vi "Check Limit&TestName Between STDF For Different Tester.vi"(7 "Result Length Array":i32[](array[numeric]), 8 "error in (no error)":errorcluster, 9 "Test Name Array":string[](array[string]), 10 "Low Limit Array":dbl[](array[numeric]), 11 "High Limit Array":dbl[](array[numeric])) -> (0 "error out":errorcluster, 3 "Test Data Out":T1)   [LabVIEW 2018, in "STDF File Parser.lvclass"]
uses:
  STDF File Parser.lvclass
  TestDataMgr/Typedefs/Test Data All.ctl
  TestDataMgr/Typedefs/Test Limits.ctl
  TestDataMgr/Typedefs/Test Raw Data.ctl
  <vilib>/Utility/error.llb/Error Cluster From Error Code.vi
  <vilib>/ErrorRing/Error Ring.xnode
  TestDataMgr/TestDataMgr.lvclass
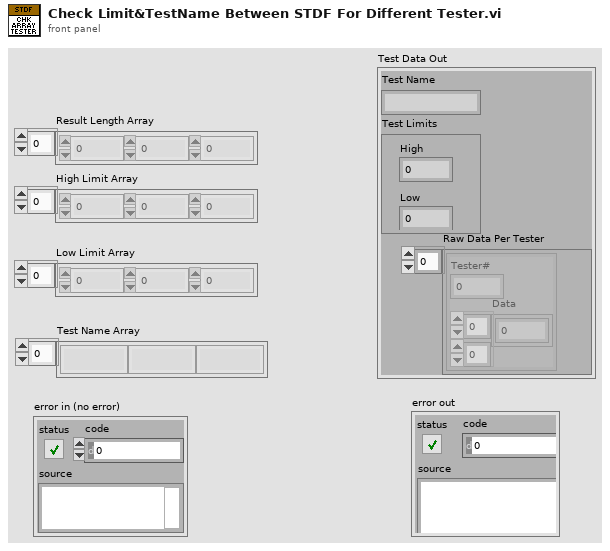
[diagram p1: front panel]
types:
  T1 = typedef "TestDataMgr.lvclass/Test Data All.ctl" = cluster{"Test Name":string, "Test Limits":T2, "Raw Data Per Tester":T3[]}
  T2 = typedef "TestDataMgr.lvclass/Test Limits.ctl" = cluster{"High":dbl, "Low":dbl}
  T3 = typedef "TestDataMgr.lvclass/Test Raw Data.ctl" = cluster{"Data":dbl[][], "Tester#":u8}
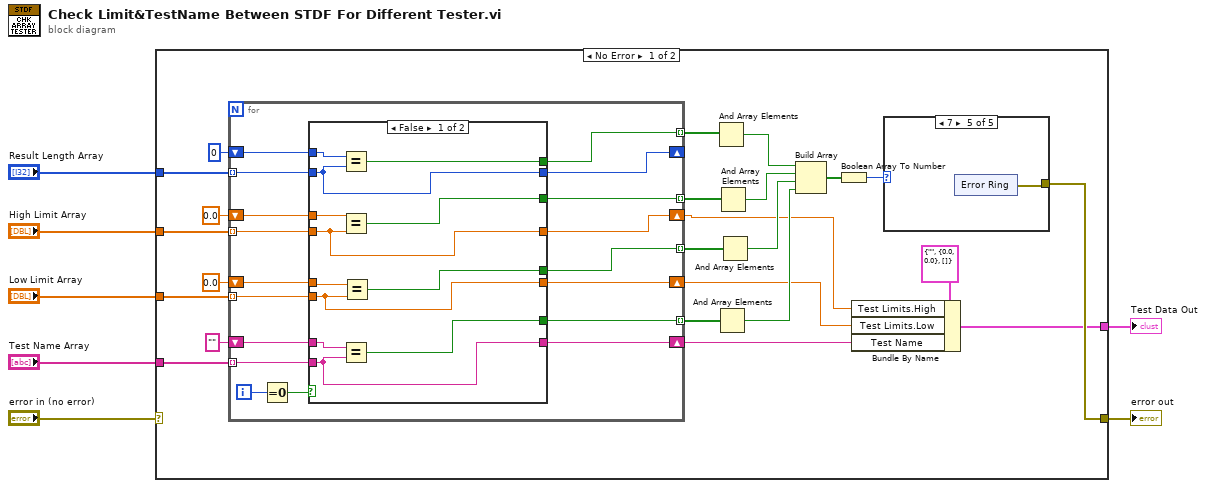
[diagram p0: block diagram]
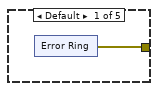
[diagram p2: hidden frame]
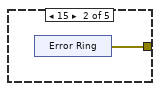
[diagram p3: hidden frame]
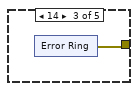
[diagram p4: hidden frame]
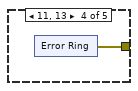
[diagram p5: hidden frame]
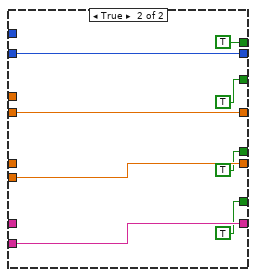
[diagram p6: hidden frame]
diagram:
  n1 = case shown="No Error" "error in (no error)" {
    selector: "error in (no error)" -> [_ w96]
    tunnel: "High Limit Array" -> [w31 _]
    tunnel: "Low Limit Array" -> [w30 _]
    tunnel: "Test Name Array" -> [w29 _]
    tunnel: "Result Length Array" -> [w25 _]
    tunnel: [w13 w96] -> w3
    tunnel: [w8 _] -> w1
    frame No Error {
      n2 = for {
        tunnel: w31 -> [w68] mode=indexing
        tunnel: w30 -> [w70] mode=indexing
        tunnel: w29 -> [w73] mode=indexing
        shift-right: [w72] -> w9
        shift-left: "" ("String") -> [w71]
        shift-right: [w69] -> w10
        shift-left: 0.0 ("High Limit Array") -> [w65]
        shift-right: [w67] -> w11
        shift-left: 0.0 ("High Limit Array") -> [w66]
        tunnel: w25 -> [w64] mode=indexing
        shift-right: [w63] -> _
        shift-left: 0 ("High Limit Array") -> [w62]
        tunnel: [w61] -> w23 mode=indexing
        tunnel: [w60] -> w22 mode=indexing
        tunnel: [w59] -> w21 mode=indexing
        tunnel: [w58] -> w20 mode=indexing
        i -> [w75]
        n3 = Equal To 0?(x=w75) -> (x = 0?=w74:bool)
        n4 = case shown="False" w74 {
          tunnel: w73 -> [w80 w95]
          tunnel: [w80 w95] -> w72
          tunnel: w71 -> [w84 _]
          tunnel: w70 -> [w81 w94]
          tunnel: [w81 w94] -> w69
          tunnel: [w82 w93] -> w67
          tunnel: w68 -> [w82 w93]
          tunnel: w66 -> [w87 _]
          tunnel: w65 -> [w85 _]
          tunnel: w64 -> [w83 w92]
          tunnel: [w83 w92] -> w63
          tunnel: w62 -> [w86 _]
          tunnel: [w79 TRUE] -> w61
          tunnel: [w76 TRUE] -> w60
          tunnel: [w78 TRUE] -> w59
          tunnel: [w77 TRUE] -> w58
          frame False {
            n5 = Equal?(x=w86, y=w83) -> (x = y?=w79:bool)
            n6 = Equal?(x=w87, y=w82) -> (x = y?=w76:bool)
            n7 = Equal?(x=w84, y=w80) -> (x = y?=w77:bool)
            n8 = Equal?(x=w85, y=w81) -> (x = y?=w78:bool)
          }
          frame True {
          }
        }
      }
      n9 = And Array Elements(Boolean array=w23) -> (logical AND=w19:bool)
      n10 = And Array Elements(Boolean array=w20) -> (logical AND=w16:bool)
      n11 = And Array Elements(Boolean array=w22) -> (logical AND=w18:bool)
      n12 = And Array Elements(Boolean array=w21) -> (logical AND=w17:bool)
      n13 = Build Array(w19, w18, w17, w16) -> (w15:bool[])
      n14 = Boolean Array To Number(Boolean array=w15) -> (number=w14:u32)
      n15 = Bundle By Name(cluster=T1 {"Test Name"="", "Test Limits"={"High"=0.0, "Low"=0.0}, "Raw Data Per Tester"=[]} ("Test Data Out"), "Test Limits.High"=w11, "Test Limits.Low"=w10, "Test Name"=w9) -> (w8:T1)
      n16 = case shown="7" w14 {
        tunnel: [w32 w38 w40 w46 w52] -> w13
        frame Default {
          n17 = xnode "Error Ring"() -> ("error out"=w32:errorcluster)
        }
        frame 15 {
          n18 = xnode "Error Ring"() -> ("error out"=w38:errorcluster)
        }
        frame 14 {
          n19 = xnode "Error Ring"() -> ("error out"=w40:errorcluster)
        }
        frame 11, 13 {
          n20 = xnode "Error Ring"() -> ("error out"=w46:errorcluster)
        }
        frame 7 {
          n21 = xnode "Error Ring"() -> ("error out"=w52:errorcluster)
        }
      }
    }
    frame Error {
    }
  }
  "error out" <- w3
  "Test Data Out" <- w1
